vi "Com_Base.vi"() -> ()   [LabVIEW 2019]
uses:
  <vilib>/Instr/_visa.llb/VISA Configure Serial Port (Instr).vi
panel:
  out "Rx Number":u8
  in  "stop":bool
  out "Receiving Data":bool
  out "Input buffer":string
  in  "Stop Acquisition":bool
  in  "VISA resource name":refnum<visa-resource-name>
  in  "Start Acquisition":bool
  # "Dades rebudes per UART"
  # "Dades transportades al Consumer Loop"
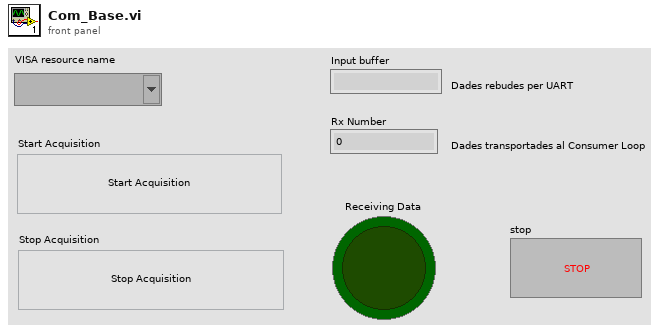
[diagram p1: front panel]
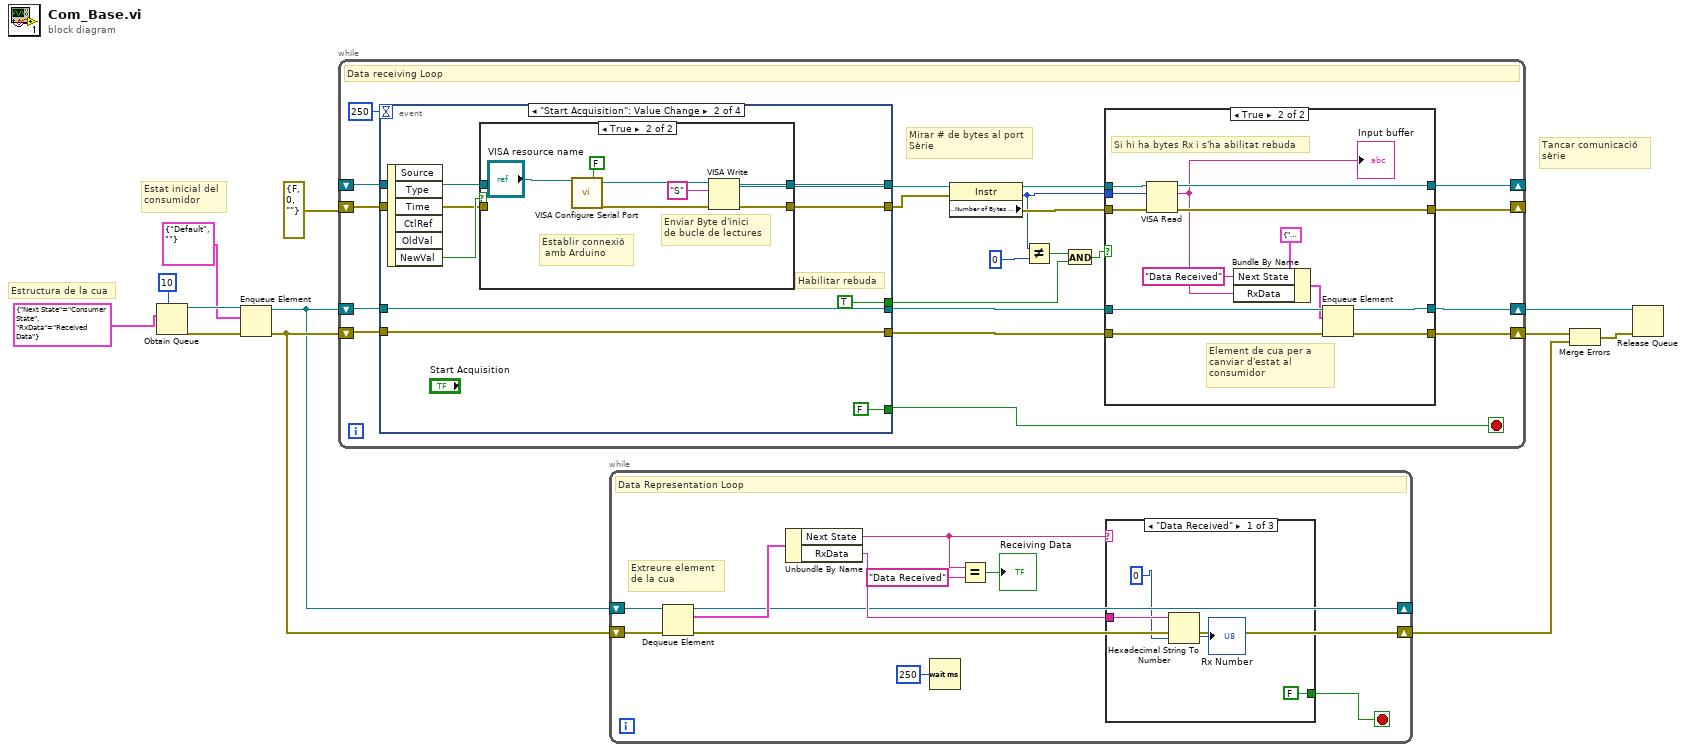
[diagram p0: block diagram]
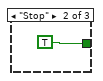
[diagram p2: hidden frame]
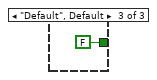
[diagram p3: hidden frame]
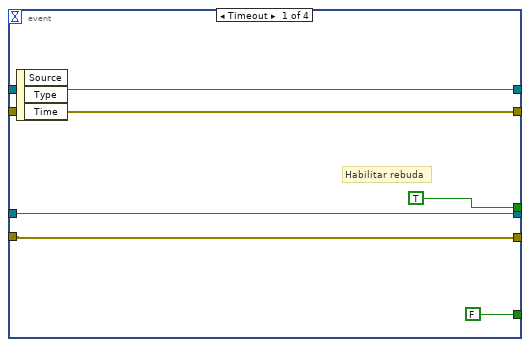
[diagram p5: hidden frame]
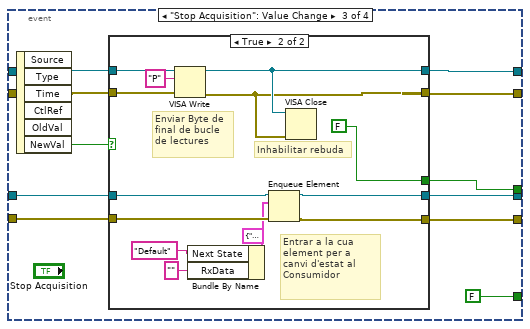
[diagram p7: hidden frame]
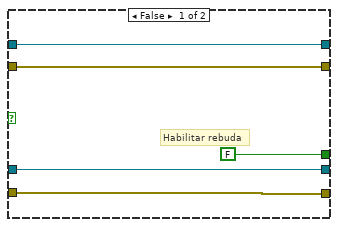
[diagram p8: hidden frame]
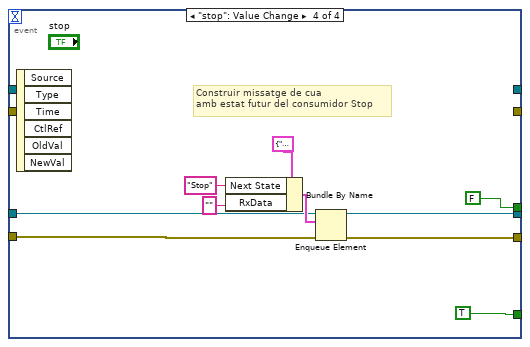
[diagram p9: hidden frame]
diagram:
  # "Estat inicial del \nconsumidor"
  # "Estructura de la cua"
  # "Tancar comunicació\nsèrie"
  n1 = Obtain Queue(max queue size (-1, unlimited)=10, element data type=cluster{"Next State":string, "RxData":string} {"Next State"="Consumer State", "RxData"="Received Data"} ("Cluster 2")) -> (queue out=w7:refnum<queue>, error out=w6:errorcluster)  [unwired: 3 in, 1 out]
  n2 = Enqueue Element(queue=w7, element=cluster{"Next State":string, "RxData":string} {"Next State"="Default", "RxData"=""} ("Cluster 2"), error in (no error)=w6) -> (queue out=w4:refnum<queue>, error out=w5:errorcluster)  [unwired: 1 in, 1 out]
  n3 = while {
    shift-right: [w33] -> _
    shift-left: _ -> [w31]
    shift-right: [w32] -> _
    shift-left: errorcluster {"status"=FALSE, "code"=0, "source"=""} ("error out") -> [w30]
    shift-right: [w27] -> w9
    shift-left: w4 -> [w17]
    shift-right: [w28] -> w11
    shift-left: w5 -> [w18]
    stop <- w13 stop-if-true
    # "Mirar # de bytes al port\nSèrie"
    # "Data receiving Loop"
    n4 = event shown="[1] \"Start Acquisition\": Value Change" {
      selector: _ -> [_ _ _ _]
      dyn-events: _ -> [_ _ _ _]
      timeout: 250 -> [_ _ _ _]
      tunnel: [w56 w65 w76 _] -> w26
      tunnel: [w55 w64 w85 _] -> w25
      tunnel: w31 -> [w56 w62 w84 _]
      tunnel: w30 -> [w55 w61 w83 _]
      tunnel: [w52 w59 w81 w107] -> w20
      tunnel: [w53 w58 w80 w106] -> w19
      tunnel: w18 -> [w53 w58 w79 w109]
      tunnel: w17 -> [w52 w59 w78 w110]
      tunnel: [TRUE TRUE w77 FALSE] -> w14
      tunnel: [FALSE FALSE FALSE TRUE] -> w13
      event Timeout {
        # "Habilitar rebuda"
        n5 = event-data() -> ()  [unwired: 1 in, 3 out]
      }
      event "Start Acquisition": Value Change {
        # "Habilitar rebuda"
        n6 = event-data() -> ("NewVal"=w63:bool)  [unwired: 1 in, 5 out]
        n7 = case shown="True" w63 {
          tunnel: [w67 w69] -> w65
          tunnel: [w66 w68] -> w64
          tunnel: w62 -> [w67 _]
          tunnel: w61 -> [w66 _]
          frame False {
          }
          frame True {
            # "Enviar Byte d'inici\nde bucle de lectures"
            # "Establir connexió\n amb Arduino"
            n8 = call-poly "VISA Configure Serial Port"("VISA resource name"="VISA resource name", "Enable Termination\nChar (T)"=FALSE ("Enable Termination\nChar (T)")) -> ("VISA resource name out"=w71:refnum<visa-resource-name>, "error out"=w72:errorcluster)  [unwired: 12 in]
            n9 = VISA Write(VISA resource name=w71, write buffer="S", error in (no error)=w72) -> (VISA resource name out=w69:refnum<visa-resource-name>, error out=w68:errorcluster)  [unwired: 1 out]
          }
        }
      }
      event "Stop Acquisition": Value Change {
        n10 = event-data() -> ("NewVal"=w82:bool)  [unwired: 1 in, 5 out]
        n11 = case shown="True" w82 {
          tunnel: [w90 w91] -> w85
          tunnel: w84 -> [w86 w104]
          tunnel: w83 -> [w90 w103]
          tunnel: [w89 w101] -> w81
          tunnel: [w88 w100] -> w80
          tunnel: w79 -> [w88 w99]
          tunnel: w78 -> [w89 w98]
          tunnel: [FALSE FALSE] -> w77
          tunnel: [w86 w92] -> w76
          frame False {
            # "Habilitar rebuda"
          }
          frame True {
            # "Entrar a la cua element per a canvi d'estat al Consumidor"
            # "Inhabilitar rebuda"
            # "Enviar Byte de \nfinal de bucle \nde lectures"
            n12 = VISA Write(VISA resource name=w104, write buffer="P", error in (no error)=w103) -> (VISA resource name out=w92:refnum<visa-resource-name>, error out=w91:errorcluster)  [unwired: 1 out]
            n13 = Bundle By Name(cluster=cluster{"Next State":string, "RxData":string} {"Next State"="", "RxData"=""} ("Cluster 2"), "Next State"="Default", "RxData"="") -> (w95:cluster{"Next State":string, "RxData":string})
            n14 = Enqueue Element(queue=w98, element=w95, error in (no error)=w99) -> (queue out=w101:refnum<queue>, error out=w100:errorcluster)  [unwired: 1 in, 1 out]
            n15 = VISA Close(VISA resource name=w92, error in (no error)=w91) -> ()  [unwired: 1 out]
          }
        }
      }
      event "stop": Value Change {
        # "Construir missatge de cua\namb estat futur del consumidor Stop"
        n16 = event-data() -> ()  [unwired: 1 in, 6 out]
        n17 = Bundle By Name(cluster=cluster{"Next State":string, "RxData":string} {"Next State"="", "RxData"=""} ("Cluster 2"), "Next State"="Stop", "RxData"="") -> (w111:cluster{"Next State":string, "RxData":string})
        n18 = Enqueue Element(queue=w110, element=w111, error in (no error)=w109) -> (queue out=w107:refnum<queue>, error out=w106:errorcluster)  [unwired: 1 in, 1 out]
      }
    }
    n19 = property class="Instr"(reference=w26, error in=w25) -> (reference out=w24:refnum<visa-resource-name>, error out=w23:errorcluster, "Serial Settings:Number of Bytes at Serial Port"=w22:u32)
    n20 = Not Equal?(x=w22, y=u32 0) -> (x != y?=w16:bool)
    n21 = And(x=w16, y=w14) -> (x .and. y?=w15:bool)
    n22 = case shown="True" w15 {
      tunnel: [w35 w50] -> w33
      tunnel: [w34 w49] -> w32
      tunnel: [w36 w48] -> w28
      tunnel: [w37 w47] -> w27
      tunnel: w19 -> [w36 w46]
      tunnel: w20 -> [w37 w45]
      tunnel: w24 -> [w35 w40]
      tunnel: w23 -> [w34 w39]
      tunnel: w22 -> [_ w38]
      frame False {
      }
      frame True {
        # "Element de cua per a canviar d'estat al consumidor"
        # "Si hi ha bytes Rx i s'ha abilitat rebuda"
        n23 = VISA Read(VISA resource name=w40, byte count=w38, error in (no error)=w39) -> (VISA resource name out=w50:refnum<visa-resource-name>, read buffer=w42:string, error out=w49:errorcluster)  [unwired: 1 out]
        "Input buffer" <- w42
        n24 = Bundle By Name(cluster=cluster{"Next State":string, "RxData":string} {"Next State"="", "RxData"=""} ("Cluster 2"), "Next State"="Data Received", "RxData"=w42) -> (w43:cluster{"Next State":string, "RxData":string})
        n25 = Enqueue Element(queue=w45, element=w43, error in (no error)=w46) -> (queue out=w47:refnum<queue>, error out=w48:errorcluster)  [unwired: 1 in, 1 out]
      }
    }
  }
  n26 = while {
    shift-right: [w122] -> w2
    shift-left: w5 -> [w124]
    shift-right: [w117] -> _
    shift-left: w4 -> [w125]
    stop <- w115 stop-if-true
    # "Extreure element \nde la cua"
    # "Data Representation Loop"
    n27 = Dequeue Element(queue=w125, error in (no error)=w124) -> (queue out=w117:refnum<queue>, element=w123:cluster{"Next State":string, "RxData":string}, error out=w122:errorcluster)  [unwired: 1 in, 1 out]
    n28 = Unbundle By Name(w123) -> ("Next State"=w120:string, "RxData"=w121:string)
    n29 = Wait (ms)(milliseconds to wait=u32 250) -> ()  [unwired: 1 out]
    n30 = Equal?(x=w120, y="Data Received") -> (x = y?=→"Receiving Data":bool)
    n31 = case shown="\"Data Received\"" w120 {
      tunnel: w121 -> [w128 _ _]
      tunnel: [FALSE TRUE FALSE] -> w115
      frame "Data Received" {
        n32 = Hexadecimal String To Number(string=w128, default (0uL)=u8 0) -> (number=→"Rx Number":u8)  [unwired: 1 in, 1 out]
      }
      frame "Stop" {
      }
      frame "Default", Default {
      }
    }
  }
  n33 = Merge Errors(w11, w2) -> (w10:errorcluster)
  n34 = Release Queue(queue=w9, error in (no error)=w10) -> ()  [unwired: 1 in, 3 out]
